vi "Parse Topic Configuration.vi"(11 "Response body":string) -> (3 "Topic Configurations":T1[](array[typedef]))   [LabVIEW 2015, in "NI_AWS_S3.lvlib"]
uses:
  NI_AWS_S3.lvlib
  Topic Configuration.ctl
  Event.ctl
  Core/HTTP Request/Name Value Pair.ctl
  XML Parsing/NI_XML Parsing.lvlib
  Core/HTTP Request/HTTP Request.lvclass
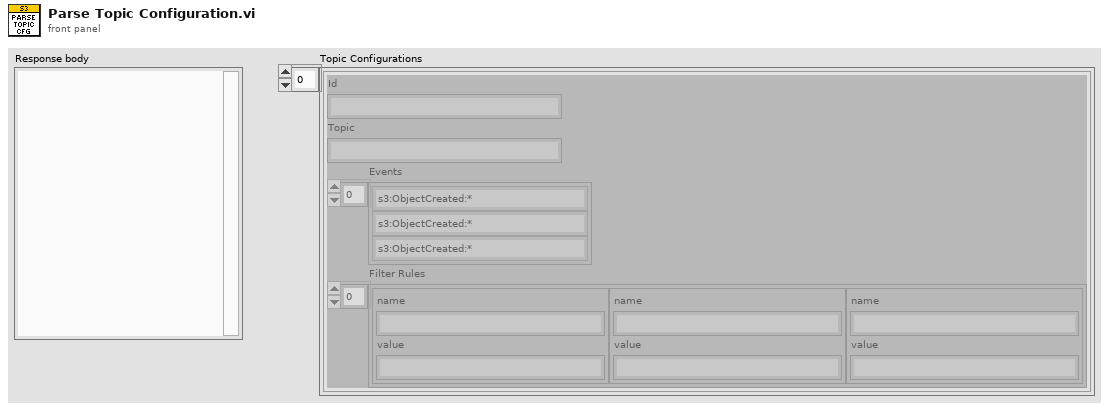
[diagram p1: front panel]
types:
  T1 = typedef "NI_AWS_S3.lvlib/Topic Configuration.ctl" = cluster{"Id":string, "Topic":string, "Events":T2[], "Filter Rules":T3[]}
  T2 = typedef "NI_AWS_S3.lvlib/Event.ctl" = enum16{"s3:ObjectCreated:*", "s3:ObjectCreated:Put", "s3:ObjectCreated:Post", "s3:ObjectCreated:Copy", "s3:ObjectCreated:CompleteMultipartUpload", "s3:ObjectRemoved:*", "s3:ObjectRemoved:Delete", "s3:ObjectRemoved:DeleteMarkerCreated", "s3:ReducedRedundancyLostObject"}
  T3 = typedef "NI_AWS_Core.lvlib/HTTP Request.lvclass/Name Value Pair.ctl" = cluster{"name":string, "value":string}
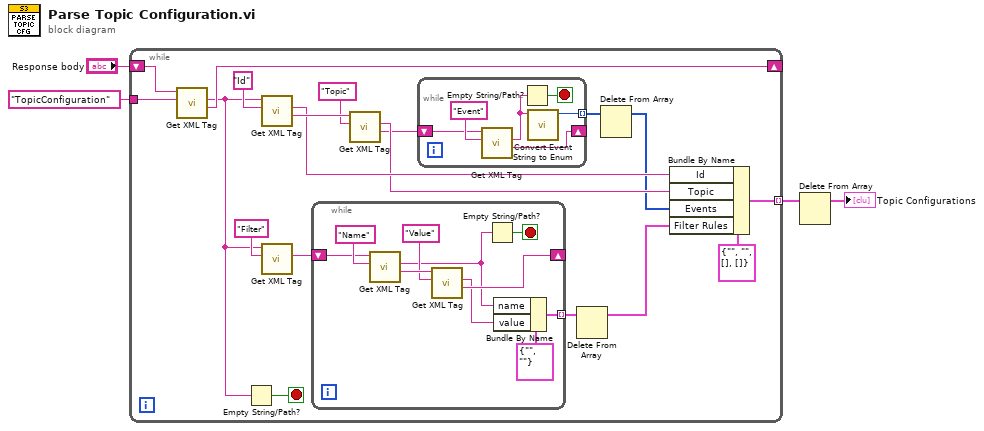
[diagram p0: block diagram]
diagram:
  n1 = while {
    shift-right: [w13] -> _
    shift-left: "Response body" -> [w23]
    tunnel: [w17] -> w3 mode=indexing
    tunnel: "TopicConfiguration" ("Tag name") -> [w5]
    stop <- w22 stop-if-true
    n2 = call "Get XML Tag.vi"("Tag name"=w5, "XML String in"=w23) -> ("Remaining string"=w13:string, "Tag value"=w8:string)  [unwired: 5 in, 3 out]
    n3 = Empty String/Path?(string/path=w8) -> (empty?=w22:bool)
    n4 = call "Get XML Tag.vi"("Tag name"="Id", "XML String in"=w8) -> ("Remaining string"=w20:string, "Tag value"=w16:string)  [unwired: 5 in, 3 out]
    n5 = call "Get XML Tag.vi"("Tag name"="Filter", "XML String in"=w8) -> ("Tag value"=w6:string)  [unwired: 5 in, 4 out]
    n6 = while {
      shift-right: [w28] -> _
      shift-left: w6 -> [w32]
      tunnel: [w24] -> w10 mode=indexing
      stop <- w31 stop-if-true
      n7 = call "Get XML Tag.vi"("Tag name"="Name", "XML String in"=w32) -> ("Remaining string"=w30:string, "Tag value"=w26:string)  [unwired: 5 in, 3 out]
      n8 = call "Get XML Tag.vi"("Tag name"="Value", "XML String in"=w30) -> ("Remaining string"=w28:string, "Tag value"=w25:string)  [unwired: 5 in, 3 out]
      n9 = Empty String/Path?(string/path=w26) -> (empty?=w31:bool)
      n10 = Bundle By Name(cluster=T3 {"name"="", "value"=""} ("FilterRule"), "name"=w26, "value"=w25) -> (w24:T3)
    }
    n11 = call "Get XML Tag.vi"("Tag name"="Topic", "XML String in"=w20) -> ("Remaining string"=w14:string, "Tag value"=w15:string)  [unwired: 5 in, 3 out]
    n12 = while {
      shift-right: [w36] -> _
      shift-left: w14 -> [w38]
      tunnel: [w37] -> w12 mode=indexing
      stop <- w35 stop-if-true
      n13 = call "Get XML Tag.vi"("Tag name"="Event", "XML String in"=w38) -> ("Remaining string"=w36:string, "Tag value"=w34:string)  [unwired: 5 in, 3 out]
      n14 = Empty String/Path?(string/path=w34) -> (empty?=w35:bool)
      n15 = call "Convert Event String to Enum.vi"("Event String"=w34) -> ("Event"=w37:T2)  [unwired: 10 in]
    }
    n16 = Delete From Array(array=w10) -> (array with subset deleted=w7:T3[])  [unwired: 2 in, 1 out]
    n17 = Delete From Array(array=w12) -> (array with subset deleted=w11:T2[])  [unwired: 2 in, 1 out]
    n18 = Bundle By Name(cluster=T1 {"Id"="", "Topic"="", "Events"=[], "Filter Rules"=[]} ("TopicConfiguration"), "Id"=w16, "Topic"=w15, "Events"=w11, "Filter Rules"=w7) -> (w17:T1)
  }
  n19 = Delete From Array(array=w3) -> (array with subset deleted=→"Topic Configurations":T1[])  [unwired: 2 in, 1 out]
